vi "连接数据库.vi"() -> (0 "error out":errorcluster, 3 "connection reference":T1)   [LabVIEW 2017]
uses:
  <vilib>/addons/database/Connection.llb/Conn ObjectReference.ctl
  <vilib>/addons/database/Connection.llb/DB Tools Open Connec (String).vi
  <vilib>/addons/database/NI_Database_API.lvlib
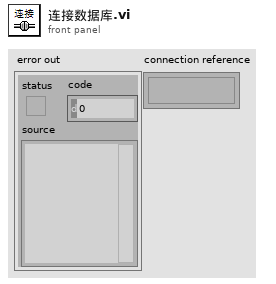
[diagram p1: front panel]
types:
  T1 = typedef "NI_Database_API.lvlib/Conn ObjectReference.ctl" = refnum<k1>
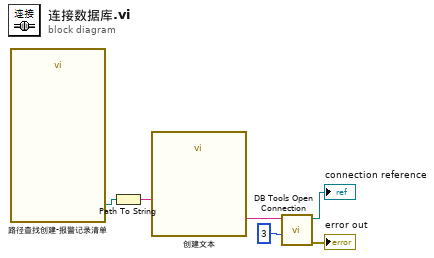
[diagram p0: block diagram]
diagram:
  n1 = call "路径查找创建-报警记录清单.vi"() -> ("数据库路径"=w4:path)  [unwired: 8 in, 11 out]
  n2 = Path To String(path=w4) -> (string=w3:string)
  n3 = call "创建文本"("文件路径"=w3) -> ("Result"=w2:string)  [unwired: 13 in, 1 out]
  n4 = call-poly <vilib>:"DB Tools Open Connection.vi"("connection timeout (15)"=3, "connection information"=w2) -> ("error out"=→"error out":errorcluster, "connection reference"=→"connection reference":T1)  [unwired: 6 in]
